vi "DFD FXP Quantize Coef.vi"   [LabVIEW 2017, in "NI_DigFilterLicensed.lvlib"]
doc: "Quantizes the coefficients of a floating-point filter and generates a fixed-point filter. You must manually select the polymorphic instance you want to use."
uses:
  <vilib>/addons/Digital Filter Design/NI_DigFilterLicensed.lvlib
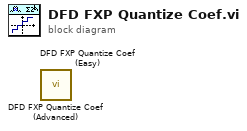
[diagram p0: block diagram]
diagram:
  n1 = call <vilib>:"DFD FXP Quantize Coef (Advanced).vi"() -> ()  [unwired: 10 in, 2 out]
  n2 = call <vilib>:"DFD FXP Quantize Coef (Easy).vi"() -> ()  [unwired: 10 in, 2 out]
